vi "D - Sort PIMHW DevList.vi"(11 "DevList":string[](array[string])) -> (1 "FE Devices":string[](array[string]), 2 "PA Devices":string[](array[string]), 3 "RF Devices":string[](array[string]))   [LabVIEW 2011]
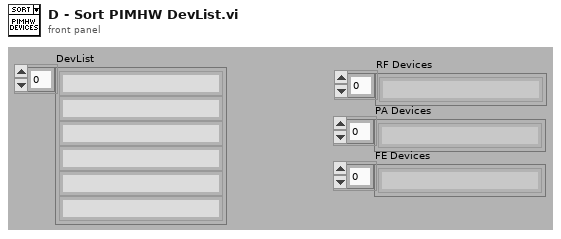
[diagram p1: front panel]
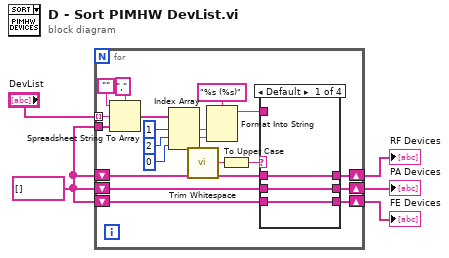
[diagram p0: block diagram]
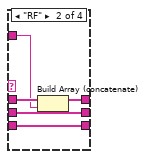
[diagram p2: hidden frame]
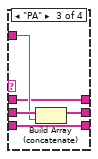
[diagram p3: hidden frame]
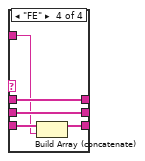
[diagram p4: hidden frame]
diagram:
  w1 = string[] [] ("DevList")
  n1 = for {
    shift-right: [w15] -> w5
    shift-left: w1 -> [w16]
    shift-right: [w12] -> w4
    shift-left: w1 -> [w14]
    shift-right: [w11] -> w3
    shift-left: w1 -> [w13]
    tunnel: "DevList" -> [w25] mode=indexing
    tunnel: w1 -> [w24]
    n2 = Spreadsheet String To Array(delimiter (Tab)=",", format string="", spreadsheet string=w25, array type (2D Dbl)=w24) -> (array=w21:string[])
    n3 = Index Array(array=w21, index #1=1 ("index"), index #2=2 ("index"), index #3=0 ("index")) -> (element #1=w19:string, element #2=w18:string, element #3=w8:string)
    n4 = call <vilib>:"Trim Whitespace.vi"("string"=w8) -> ("trimmed string"=w9:string)  [unwired: 1 in]
    n5 = Format Into String(format string="%s (%s)", w19, w18) -> (resulting string=w17:string)  [unwired: 2 in, 1 out]
    n6 = To Upper Case(1:w9) -> (0:w7:string)
    n7 = case shown="Default" w7 {
      tunnel: w17 -> [_ w33 w37 w40]
      tunnel: w16 -> [w29 w34 w36 w42]
      tunnel: [w29 w32 w36 w42] -> w15
      tunnel: w14 -> [w28 w31 w39 w41]
      tunnel: w13 -> [w27 w30 w35 w44]
      tunnel: [w28 w31 w38 w41] -> w12
      tunnel: [w27 w30 w35 w43] -> w11
      frame Default {
      }
      frame "RF" {
        n8 = Build Array (concatenate)(w34, w33) -> (w32:string[])
      }
      frame "PA" {
        n9 = Build Array (concatenate)(w39, w37) -> (w38:string[])
      }
      frame "FE" {
        n10 = Build Array (concatenate)(w44, w40) -> (w43:string[])
      }
    }
  }
  "RF Devices" <- w5
  "PA Devices" <- w4
  "FE Devices" <- w3
